vi "TDC_getChannelDelays.vi"(8 "Error In":errorcluster) -> (0 "Error Out":errorcluster)   [LabVIEW 2011]
uses:
  tdcbase.dll
panel:
  out "Delays":i32[](array[numeric])
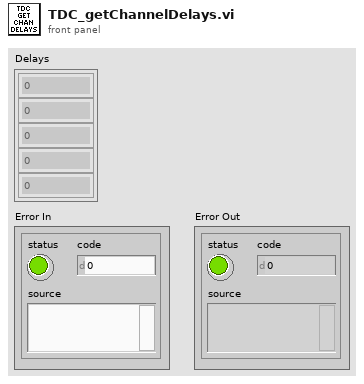
[diagram p1: front panel]
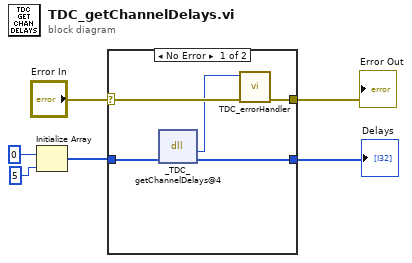
[diagram p0: block diagram]
diagram:
  n1 = Initialize Array(0, 5) -> (w1:i32[])
  n2 = case shown="No Error" "Error In" {
    selector: "Error In" -> [w10 w13]
    tunnel: [w9 w13] -> w5
    tunnel: [w11 w12] -> w4
    tunnel: w1 -> [w7 w12]
    frame No Error {
      n3 = dll-call lib="X:/tdcbase.dll" fn="_TDC_getChannelDelays@4"("delays"=w7) -> ("return type"=w8:i32, "delays"=w11:i32[])  [unwired: 3 in, 2 out]
      n4 = call "TDC_errorHandler.vi"("Error In"=w10, "TDC Return Code"=w8) -> ("Error Out"=w9:errorcluster)  [unwired: 9 in]
    }
    frame Error {
    }
  }
  "Error Out" <- w5
  "Delays" <- w4
